vi "Co-Pilot_drive_filter.vi"(11 "Co-Pilot Data":T1) -> (3 "output cluster":T1)   [LabVIEW 2014]
uses:
  Co-Pilot_game_control.ctl
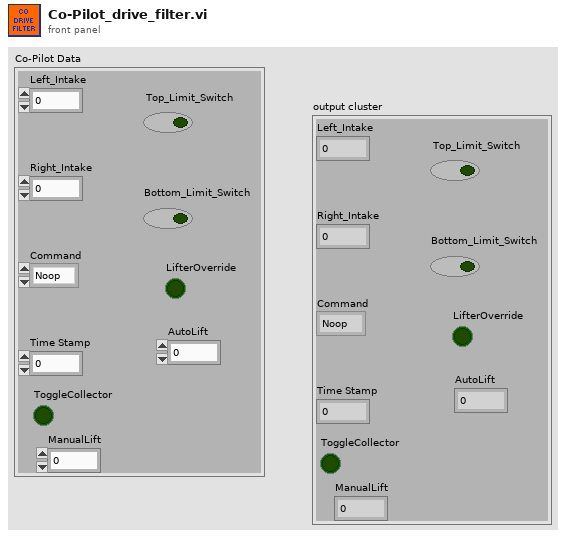
[diagram p1: front panel]
types:
  T1 = typedef "Co-Pilot_game_control.ctl" = cluster{"Left_Intake":dbl, "Right_Intake":dbl, "Time Stamp":u32, "Command":enum16{"Noop", "Flagged"}, "ToggleCollector":bool, "ManualLift":dbl, "Top_Limit_Switch":bool, "Bottom_Limit_Switch ":bool, "LifterOverride":bool, "AutoLift":i32}
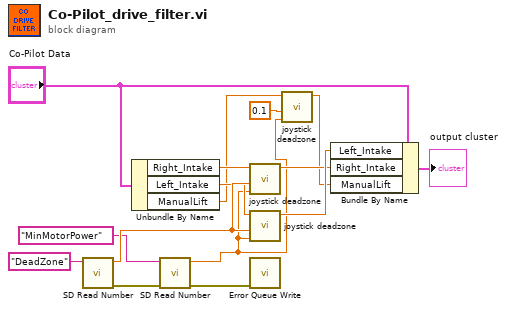
[diagram p0: block diagram]
diagram:
  n1 = call <vilib>:"SD Read Number.vi"("Name"="DeadZone") -> ("error out"=w9:errorcluster, "Numeric"=w13:dbl)  [unwired: 8 in, 1 out]
  n2 = Unbundle By Name("Co-Pilot Data") -> ("Right_Intake"=w12:dbl, "Left_Intake"=w11:dbl, "ManualLift"=w3:dbl)
  n3 = call <vilib>:"SD Read Number.vi"("error in"=w9, "Name"="MinMotorPower") -> ("error out"=w10:errorcluster, "Numeric"=w1:dbl)  [unwired: 7 in, 1 out]
  n4 = call "joystick deadzone.vi"("minpower"=w1, "deadzone"=w13, "joystick"=w12) -> ("joyout"=w14:dbl)  [unwired: 8 in]
  n5 = call "joystick deadzone.vi"("minpower"=w1, "deadzone"=w13, "joystick"=w11) -> ("joyout"=w15:dbl)  [unwired: 8 in]
  n6 = call "Error Queue Write.vi"("error in (no error)"=w10) -> ()  [unwired: 11 in]
  n7 = call "joystick deadzone.vi"("minpower"=w1, "deadzone"=0.1, "joystick"=w3) -> ("joyout"=w4:dbl)  [unwired: 8 in]
  n8 = Bundle By Name(cluster="Co-Pilot Data", "Left_Intake"=w15, "Right_Intake"=w14, "ManualLift"=w4) -> (→"output cluster":T1)
